vi "Keep Min.vi"(7 "Reset(F)":bool, 11 "Value":dbl) -> (3 "min":dbl)   [LabVIEW 2017]
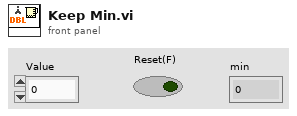
[diagram p1: front panel]
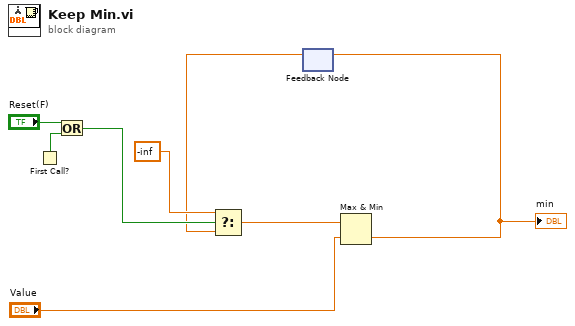
[diagram p0: block diagram]
diagram:
  n1 = First Call?() -> (First Call?: T/F=w7:bool)
  n2 = Or(x="Reset(F)", y=w7) -> (x .or. y?=w6:bool)
  n3 = feedback #1() -> (w2:dbl)  [unwired: 1 in]
  n4 = Select(t=-inf, s=w6, f=w2) -> (s? t:f=w4:dbl)
  n5 = Max & Min(x=w4, y="Value") -> (min(x,y)=w1:dbl)  [unwired: 1 out]
  "min" <- w1
  n6 = feedback-in #1(w1) -> ()
